vi "Get Bmp Color Table.vi"(8 "错误输入":errorcluster, 9 "Offset":i32, 10 "Info Header In":T1, 11 "Bmp Data In":string) -> (0 "错误输出":errorcluster, 1 "Offset":i32, 2 "Info Header Out":T1, 3 "Bmp Data Out":string, 5 "Color Table":u32[](array[numeric]))   [LabVIEW 2011, in "BMP File.lvlib"]
uses:
  BMP File.lvlib
  Bmp Info Header.ctl
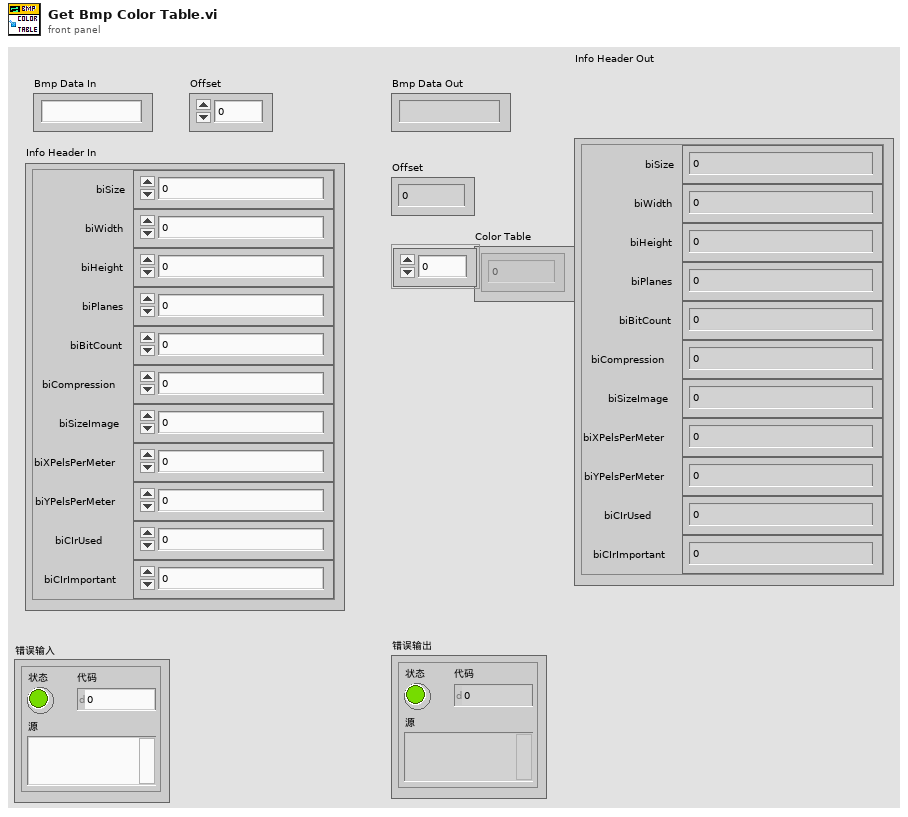
[diagram p1: front panel]
types:
  T1 = typedef "BMP File.lvlib/Bmp Info Header.ctl" = cluster{"biSize":u32, "biWidth":i32, "biHeight":i32, "biPlanes":u16, "biBitCount":u16, "biCompression":u32, "biSizeImage":u32, "biXPelsPerMeter":i32, "biYPelsPerMeter":i32, "biCIrUsed":u32, "biCIrImportant":u32}
  T2 = enum16{"big-endian, network order", "native, host order", "little-endian"}
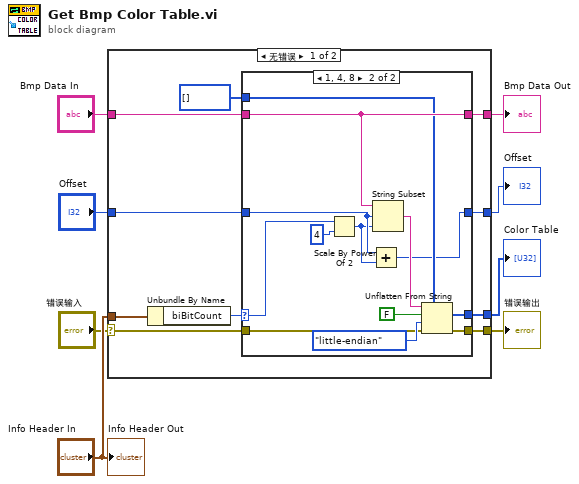
[diagram p0: block diagram]
diagram:
  n1 = case shown="无错误" "错误输入" {
    selector: "错误输入" -> [w14 w38]
    tunnel: "Info Header In" -> [w18 _]
    tunnel: "Bmp Data In" -> [w17 w36]
    tunnel: "Offset" -> [w16 w37]
    tunnel: [w13 w38] -> w4
    tunnel: [w11 _] -> w3
    tunnel: [w10 w37] -> w2
    tunnel: [w9 w36] -> w1
    frame No Error {
      n2 = Unbundle By Name(w18) -> ("biBitCount"=w15:u16)
      n3 = case shown="1, 4, 8" w15 {
        selector: w15 -> [_ w35]
        tunnel: w17 -> [w22 w33]
        tunnel: w16 -> [w19 w26]
        tunnel: [w22 w33] -> w9
        tunnel: w14 -> [w21 w30]
        tunnel: [w21 w29] -> w13
        tunnel: u32[] [] -> [w20 w28]
        tunnel: [w20 w27] -> w11
        tunnel: [w19 w24] -> w10
        frame 0, Default {
        }
        frame 1, 4, 8 {
          n4 = Scale By Power Of 2(n=w35, x=u16 4 ("biBitCount")) -> (x*2^n=w25:u16)
          n5 = Add(x=w26, y=w25) -> (x+y=w24:i32)
          n6 = String Subset(string=w33, offset (0)=w26, length (rest)=w25) -> (substring=w32:string)
          n7 = Unflatten From String(type=w28, binary string=w32, data includes array or string size? (T)=FALSE ("数据中包含数组或字符串大小？(T)"), byte order (0:big-endian, network order)=T2."little-endian" ("字节顺序(0:big-endian, network order)"), error in (no error)=w30) -> (value=w27:u32[], error out=w29:errorcluster)  [unwired: 1 out]
        }
      }
    }
    frame Error {
    }
  }
  "错误输出" <- w4
  "Color Table" <- w3
  "Offset" <- w2
  "Bmp Data Out" <- w1
  "Info Header Out" <- "Info Header In"
